vi "QueuedStateMachine with Error Handler.vi"(8 "ErrI":errorcluster) -> (0 "ErrO":errorcluster)   [LabVIEW 2020]
panel:
  in  "Exit":bool
  in  "OK":bool
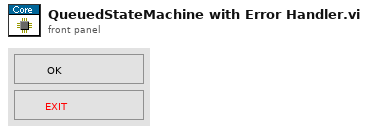
[diagram p1: front panel]
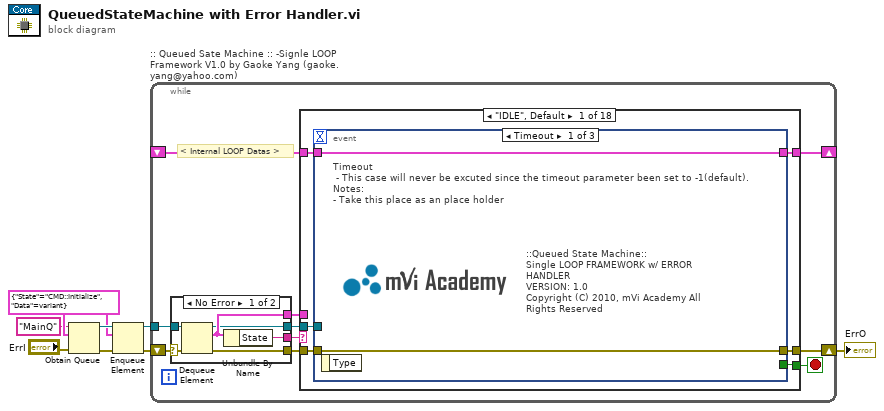
[diagram p0: block diagram]
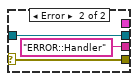
[diagram p2: hidden frame]
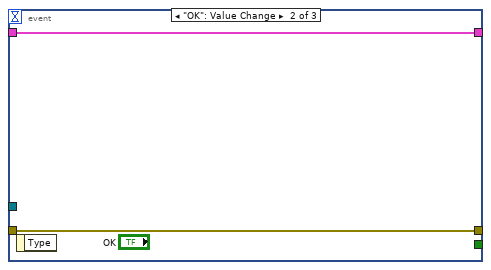
[diagram p3: hidden frame]
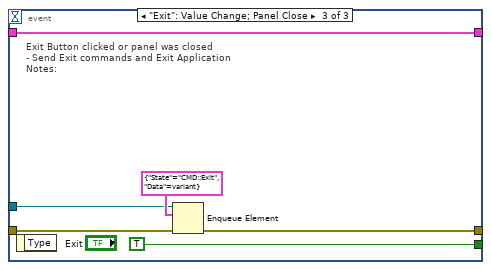
[diagram p4: hidden frame]
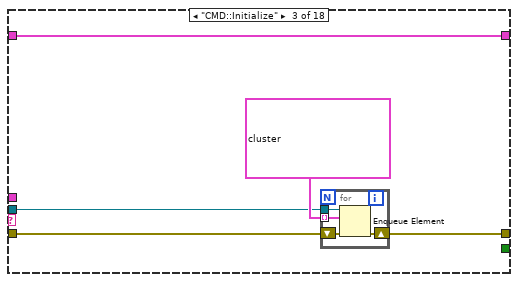
[diagram p6: hidden frame]
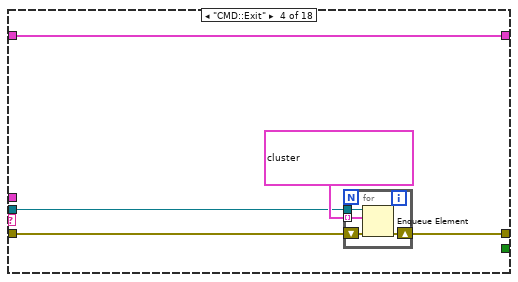
[diagram p7: hidden frame]
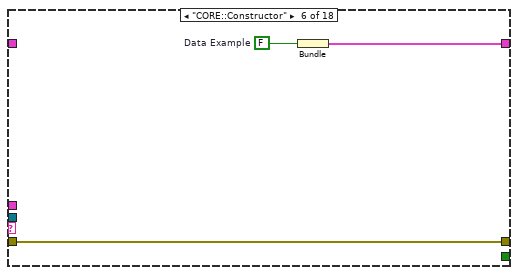
[diagram p9: hidden frame]
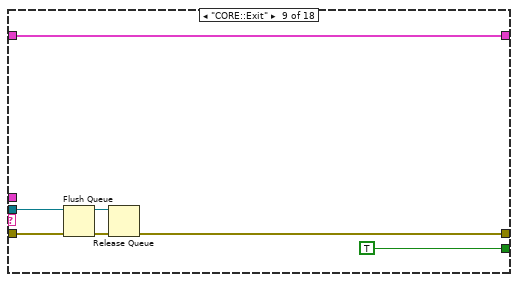
[diagram p12: hidden frame]
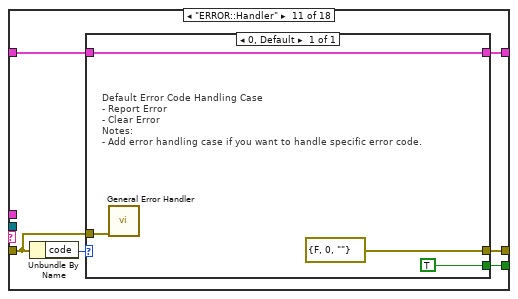
[diagram p14: hidden frame]
diagram:
  w6 = cluster{"State":string, "Data":variant} {"State"="CMD::Initialize", "Data"=variant} ("MainQueue")
  n1 = Obtain Queue(name (unnamed)="MainQ", element data type=w6, error in (no error)="ErrI") -> (queue out=w8:refnum<queue>, error out=w7:errorcluster)  [unwired: 2 in, 1 out]
  n2 = Enqueue Element(queue=w8, element=w6, error in (no error)=w7) -> (queue out=w4:refnum<queue>, error out=w3:errorcluster)  [unwired: 2 out]
  n3 = while ":: Queued Sate Machine :: -Signle LOOP Framework V1.0 by Gaoke Yang (gaoke.yang@yahoo.com)" {
    tunnel: w4 -> [w11]
    shift-right: [w10] -> w1
    shift-left: w3 -> [w12]
    shift-right: [w14] -> _
    shift-left: _ -> [w13]
    stop <- w17 stop-if-true
    # "< Internal LOOP Datas >"
    n4 = case shown="No Error" w12 {
      selector: w12 -> [w20 w27]
      tunnel: w11 -> [w24 w25]
      tunnel: [w23 w27] -> w18
      tunnel: [w22 "ERROR::Handler" ("State")] -> w16
      tunnel: [w21 _] -> w15
      tunnel: [w19 w25] -> w9
      frame No Error {
        n5 = Dequeue Element(queue=w24, error in (no error)=w20) -> (queue out=w19:refnum<queue>, element=w21:cluster{"State":string, "Data":variant}, error out=w23:errorcluster)  [unwired: 2 out]
        n6 = Unbundle By Name(w21) -> ("State"=w22:string)
      }
      frame Error {
      }
    }
    n7 = case shown="\"IDLE\", Default" w16 {
      tunnel: [w30 w45 w49 w58 w65 w68 w70 w72 w74 w81 w84 w92 w94 w96 w99 w101 w103 w104] -> w10
      tunnel: [w29 _ _ _ _ _ _ _ TRUE _ w83 _ _ _ _ _ _ _] -> w17
      tunnel: w18 -> [w31 w45 w48 w57 w65 w68 w70 w72 w78 w81 w82 w92 w94 w96 w99 w101 w103 w104]
      tunnel: w15 -> [_ _ _ _ _ _ _ _ _ _ _ _ _ _ _ _ _ _]
      tunnel: [w32 w44 w50 w59 w64 w66 w69 w71 w76 w80 w85 w93 w95 w97 w98 w100 w102 w105] -> w14
      tunnel: w13 -> [w33 w44 w50 w59 w64 _ w69 w71 w76 w80 w86 w93 w95 w97 w98 w100 w102 w105]
      tunnel: w9 -> [w28 _ w46 w55 _ _ _ _ w73 _ _ _ _ _ _ _ _ _]
      frame "IDLE", Default {
        n8 = event shown="[0] Timeout" {
          selector: _ -> [_ _ _]
          dyn-events: _ -> [_ _ _]
          timeout: _ -> [_ _ _]
          tunnel: [_ _ TRUE ("Exit")] -> w29
          tunnel: w31 -> [w35 w37 w40]
          tunnel: [w35 w37 w41] -> w30
          tunnel: [w34 w36 w43] -> w32
          tunnel: w33 -> [w34 w36 w43]
          tunnel: w28 -> [_ _ w38]
          event Timeout {
            # "Timeout\n - This case will never be excuted since the timeout parameter been set to -1(default).\nNotes:\n- Take this place as an place holder"
            # "::Queued State Machine::\nSingle LOOP FRAMEWORK w/ ERROR HANDLER\nVERSION: 1.0\nCopyright (C) 2010, mVi Academy All Rights Reserved"
            n9 = event-data() -> ()  [unwired: 2 out]
          }
          event "OK": Value Change {
            n10 = event-data() -> ()  [unwired: 2 out]
          }
          event "Exit": Value Change; Panel Close {
            # "Exit Button clicked or panel was closed\n- Send Exit commands and Exit Application\nNotes:"
            n11 = event-data() -> ()  [unwired: 2 out]
            n12 = Enqueue Element(queue=w38, element=cluster{"State":string, "Data":variant} {"State"="CMD::Exit", "Data"=variant} ("MainQueue"), error in (no error)=w40) -> (error out=w41:errorcluster)  [unwired: 3 out]
          }
        }
      }
      frame "-------- Commands ---------" {
      }
      frame "CMD::Initialize" {
        n13 = for {
          shift-right: [w53] -> w49
          shift-left: w48 -> [w54]
          tunnel: cluster{"State":string, "Data":variant}[] [{"State"="CORE::Constructor", "Data"=variant}, {"State"="CORE::Initialize", "Data"=variant}, {"State"="IDLE", "Data"=variant}] -> [w52] mode=indexing
          tunnel: w46 -> [w51]
          n14 = Enqueue Element(queue=w51, element=w52, error in (no error)=w54) -> (error out=w53:errorcluster)  [unwired: 3 out]
        }
      }
      frame "CMD::Exit" {
        n15 = for {
          shift-right: [w62] -> w58
          shift-left: w57 -> [w63]
          tunnel: cluster{"State":string, "Data":variant}[] [{"State"="CORE::DeConstructor", "Data"=variant}, {"State"="CORE::Exit", "Data"=variant}] -> [w61] mode=indexing
          tunnel: w55 -> [w60]
          n16 = Enqueue Element(queue=w60, element=w61, error in (no error)=w63) -> (error out=w62:errorcluster)  [unwired: 3 out]
        }
      }
      frame "------------ Core ------------" {
      }
      frame "CORE::Constructor" {
        w67 = FALSE  # Data Example
        n17 = Bundle("Data Example"=w67) -> (w66:cluster{"Data Example":bool})  [unwired: 1 in]
      }
      frame "CORE::Initialize" {
      }
      frame "CORE::DeConstructor" {
      }
      frame "CORE::Exit" {
        n18 = Flush Queue(queue=w73, error in (no error)=w78) -> (queue out=w75:refnum<queue>, error out=w77:errorcluster)  [unwired: 1 out]
        n19 = Release Queue(queue=w75, error in (no error)=w77) -> (error out=w74:errorcluster)  [unwired: 1 in, 2 out]
      }
      frame "-------- Error Handle--------" {
      }
      frame "ERROR::Handler" {
        n20 = Unbundle By Name(w82) -> ("code"=w87:i32)
        n21 = case shown="0, Default" w87 {
          tunnel: [w91] -> w85
          tunnel: w86 -> [w91]
          tunnel: [errorcluster {"status"=FALSE, "code"=0, "source"=""} ("error out")] -> w84
          tunnel: [TRUE] -> w83
          tunnel: w82 -> [w89]
          frame 0, Default {
            # "Default Error Code Handling Case\n- Report Error\n- Clear Error \nNotes:\n- Add error handling case if you want to handle specific error code."
            n22 = call <vilib>:"General Error Handler.vi"("error in (no error)"=w89) -> ()  [unwired: 10 in, 5 out]
          }
        }
      }
      frame "------------  GUI  ------------" {
      }
      frame "GUI::Initialize" {
      }
      frame "GUI::SetCusor" {
      }
      frame "GUI::SetMenu" {
      }
      frame "------------ USER -----------" {
      }
      frame "USER::Case1" {
      }
      frame "USER::Case2" {
      }
    }
  }
  "ErrO" <- w1
